vi "Publish Element.vi"(8 "Timeout mS (-1)":i32, 9 "element":T1, 11 "Channel Data In":T2) -> (1 "Closed":bool, 2 "Timeout":bool)   [LabVIEW 2020, in "Flex.lvlib"]
uses:
  Flex.lvlib
  Element.ctl
  Channel Data.ctl
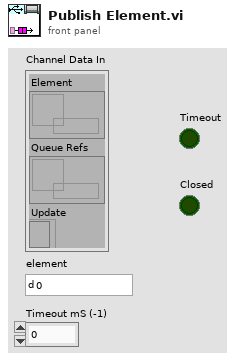
[diagram p1: front panel]
types:
  T1 = typedef "Flex.lvlib/Element.ctl" = dbl
  T2 = typedef "Flex.lvlib/Channel Data.ctl" = cluster{"Element":refnum<data-value>, "Queue Refs":refnum<data-value>, "Update":refnum<k4>}
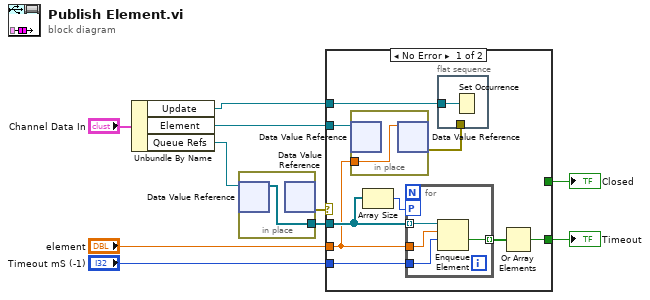
[diagram p0: block diagram]
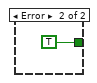
[diagram p2: hidden frame]
diagram:
  n1 = Unbundle By Name("Channel Data In") -> ("Update"=w2:refnum<k4>, "Element"=w3:refnum<data-value>, "Queue Refs"=w9:refnum<data-value>)
  n2 = in-place {
    in-place-border: [w11] -> w8
    n3 = in-place-dvr #1(w9) -> (w11:refnum<queue>[])  [unwired: 1 out]
    n4 = in-place-dvr #1() -> (w4:errorcluster)  [unwired: 1 in, 1 out]
  }
  n5 = case shown="No Error" w4 {
    tunnel: w8 -> [w19 _]
    tunnel: "Timeout mS (-1)" -> [w18 _]
    tunnel: "element" -> [w14 _]
    tunnel: [w16 _] -> w5
    tunnel: w3 -> [w15 _]
    tunnel: w2 -> [w13 _]
    tunnel: [_ TRUE] -> w1
    frame No Error {
      n6 = in-place {
        in-place-border: w14 -> [w22]
        n7 = in-place-dvr #2(w15) -> ()  [unwired: 2 out]
        n8 = in-place-dvr #2(w22) -> (w12:errorcluster)  [unwired: 1 out]
      }
      n9 = Array Size(array=w19) -> (size(s)=w20:i32)
      n10 = for {
        workers-P: w20 -> [_]
        tunnel: w19 -> [w26] mode=indexing
        tunnel: w18 -> [w25]
        tunnel: w14 -> [w24]
        tunnel: [w23] -> w17 mode=indexing
        n11 = Enqueue Element(queue=w26, element=w24, timeout in ms (-1)=w25) -> (timed out?=w23:bool)  [unwired: 1 in, 2 out]
      }
      n12 = flat-sequence {
        tunnel: w13 -> [w21]
        tunnel: w12 -> [_]
        frame #0 {
          n13 = Set Occurrence(w21) -> ()
        }
      }
      n14 = Or Array Elements(Boolean array=w17) -> (logical OR=w16:bool)
    }
    frame Error {
    }
  }
  "Timeout" <- w5
  "Closed" <- w1
